vi "cam_example.vi"() -> ()   [LabVIEW 2020]
uses:
  <vilib>/userdefined/High Color/IMAQdx.ctl
  <vilib>/vision/driver/NI_Vision_Acquisition_Software.lvlib
  <resource>/objmgr/imaqdx.rc
  source/repos/cont2019/x64/Release/Image_processing.dll
panel:
  in  "Num frames":i32=3
  out "maximum":u8
  out "FPS":dbl
  in  "Exposure time":dbl=1000.0
  out "Power":dbl(graph)
  out "Image":T1(plugin-control)
  in  "stop":bool
  in  "Session In":T2="cam2"
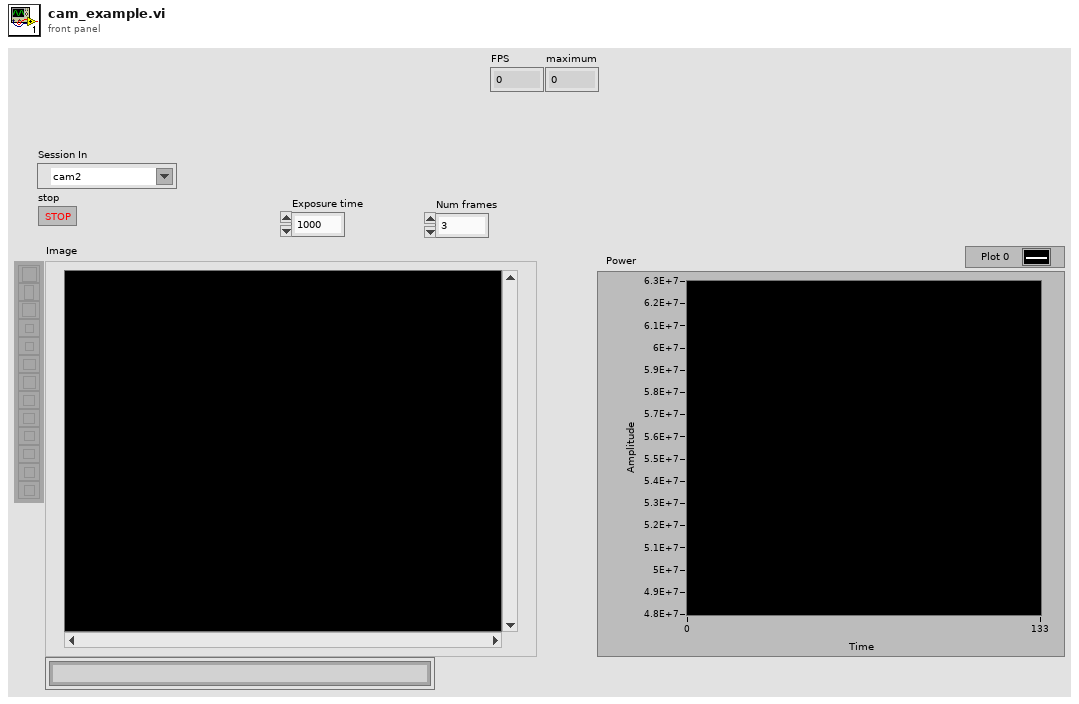
[diagram p1: front panel]
types:
  T1 = typedef "IMAQ Image.ctl" = refnum<image>
  T2 = typedef "IMAQdx.ctl" = refnum<k21>
  T3 = cluster{"Global Rectangle":i32[], "Contours":cluster{"Contour Type":u32, "ROI Type":u32, "Points":i32[]}[]}
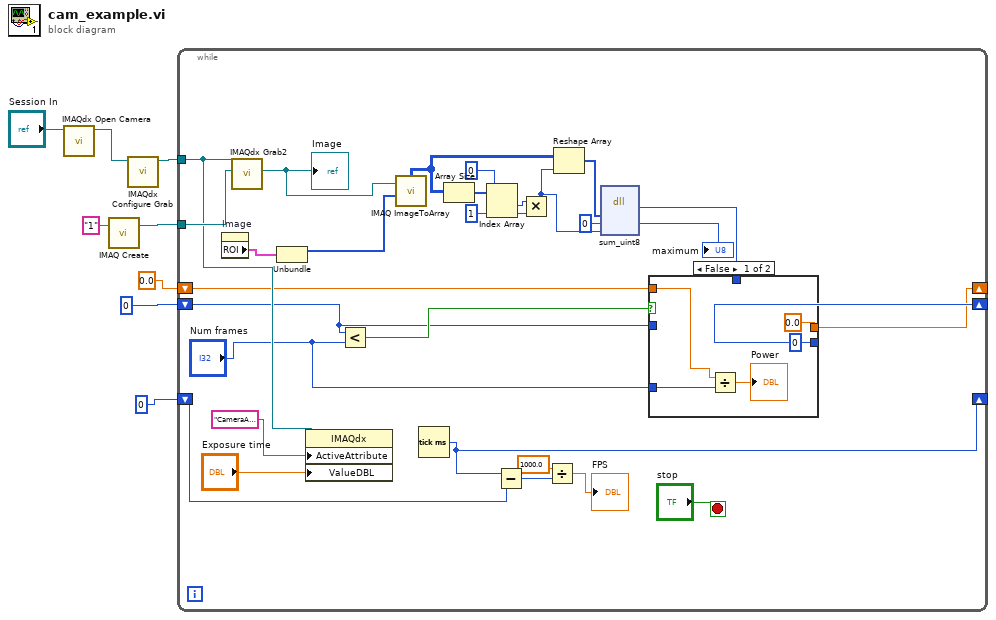
[diagram p0: block diagram]
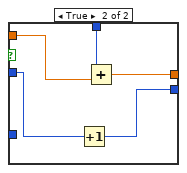
[diagram p2: hidden frame]
diagram:
  n1 = call <vilib>:"IMAQdx Open Camera.vi"("Session In"="Session In") -> ("Session Out"=w7:T2)  [unwired: 9 in, 1 out]
  n2 = call "IMAQ Create"("Image Name"="1") -> ("New Image"=w4:T1)  [unwired: 4 in, 1 out]
  n3 = call <vilib>:"IMAQdx Configure Grab.vi"("Session In"=w7) -> ("Session Out"=w6:T2)  [unwired: 9 in, 1 out]
  n4 = while {
    tunnel: w6 -> [w20]
    tunnel: w4 -> [w27]
    shift-right: [w25] -> _
    shift-left: 0 -> [w26]
    shift-right: [w14] -> _
    shift-left: 0 -> [w15]
    shift-right: [w10] -> _
    shift-left: 0.0 -> [w12]
    stop <- "stop" stop-if-true
    n5 = property on="Image" class="ImageControl"() -> ("ROI"=w36:T3)  [unwired: 2 in, 2 out]
    n6 = call <vilib>:"IMAQdx Grab2.vi"("Image In"=w27, "Session In"=w20) -> ("Image Out"=w37:T1)  [unwired: 6 in, 3 out]
    "Image" <- w37
    n7 = Unbundle(w36) -> ("Global Rectangle"=w35:i32[])  [unwired: 1 out]
    n8 = property class="IMAQdx"(reference=w20, "ActiveAttribute"="CameraAttributes::AcquisitionControl::ExposureTime" ("ValueString"), "ValueDBL"="Exposure time") -> ()  [unwired: 1 in, 2 out]
    n9 = Less?(x=w15, y="Num frames") -> (x < y?=w16:bool)
    n10 = call "IMAQ ImageToArray"("Optional Rectangle"=w35, "Image"=w37) -> ("Image Pixels (U8)"=w29:u8[][])  [unwired: 2 in, 4 out]
    n11 = Tick Count (ms)() -> (millisecond timer value=w25:u32)
    n12 = Array Size(array=w29) -> (size(s)=w34:i32[])
    n13 = Index Array(array=w34, index #1=0 ("index"), index #2=1 ("index")) -> (element #1=w31:i32, element #2=w30:i32)
    n14 = Subtract(x=w25, y=w26) -> (x-y=w22:u32)
    n15 = Multiply(x=w31, y=w30) -> (x*y=w28:i32)
    n16 = Divide(x=1000.0, y=w22) -> (x/y=→"FPS":dbl)
    n17 = Reshape Array(w29, w28) -> (w18:u8[])
    n18 = dll-call lib="C:/Users/lenovo/source/repos/cont2019/x64/Release/Image_processing.dll" fn="sum_uint8"("pixel_data"=w18, "maximum"=u8 0, "lenght"=w28) -> ("sum"=w11:u64, "maximum"=→"maximum":u8)  [unwired: 5 in, 2 out]
    n19 = case shown="False" w16 {
      tunnel: w15 -> [_ w48]
      tunnel: [0 w47] -> w14
      tunnel: w12 -> [w40 w46]
      tunnel: w11 -> [_ w45]
      tunnel: [0.0 w44] -> w10
      tunnel: "Num frames" -> [w39 _]
      frame False {
        n20 = Divide(x=w40, y=w39) -> (x/y=→"Power":dbl)
      }
      frame True {
        n21 = Increment(x=w48) -> (x+1=w47:i32)
        n22 = Add(x=w45, y=w46) -> (x+y=w44:dbl)
      }
    }
  }
